vi "Mexa_7170 - 3.vi"(0 "String 1 In":string, 1 "Connect":bool, 2 "IP Array":string[](array[string]), 5 "connection ID 1 In":refnum<k5>, 7 "error out 1 In":errorcluster, 9 "connection ID 2 In":refnum<k16>, 11 "error out 2 In":errorcluster, 12 "Time In":i16) -> (3 "Emissions":dbl[](array[numeric]), 4 "String 1 Out":string, 6 "connection ID 1 Out":refnum<k5>, 8 "error 1 out":errorcluster, 10 "connection ID 2 Out":refnum<k16>, 14 "Time Out":i16, 15 "error 2 out":errorcluster)   [LabVIEW 2014]
panel:
  in  "stop":bool
  out "Array out":dbl[](array[numeric])
  in  "stop TCP 2":bool
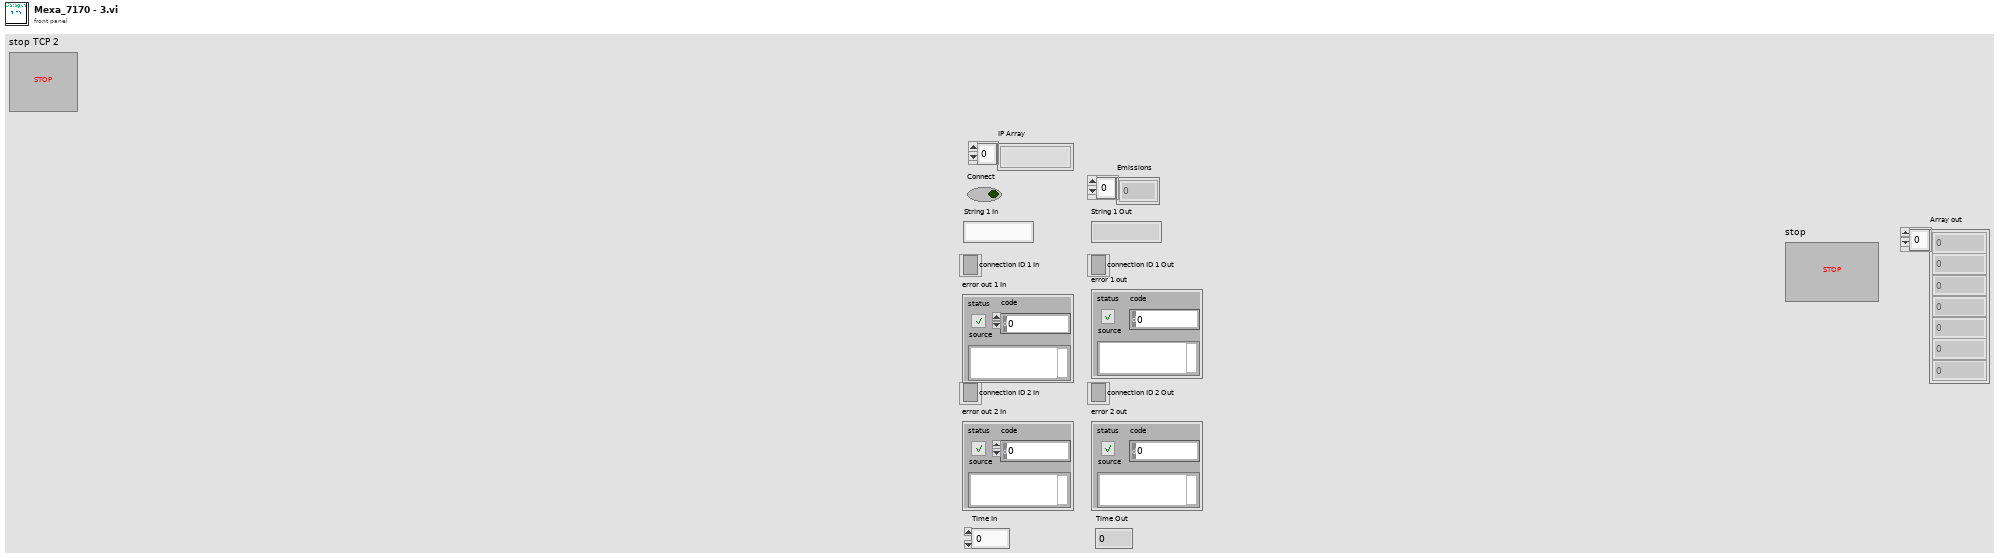
[diagram p1: front panel]
types:
  T1 = cluster{"status":bool, "code":bool, "source":bool}
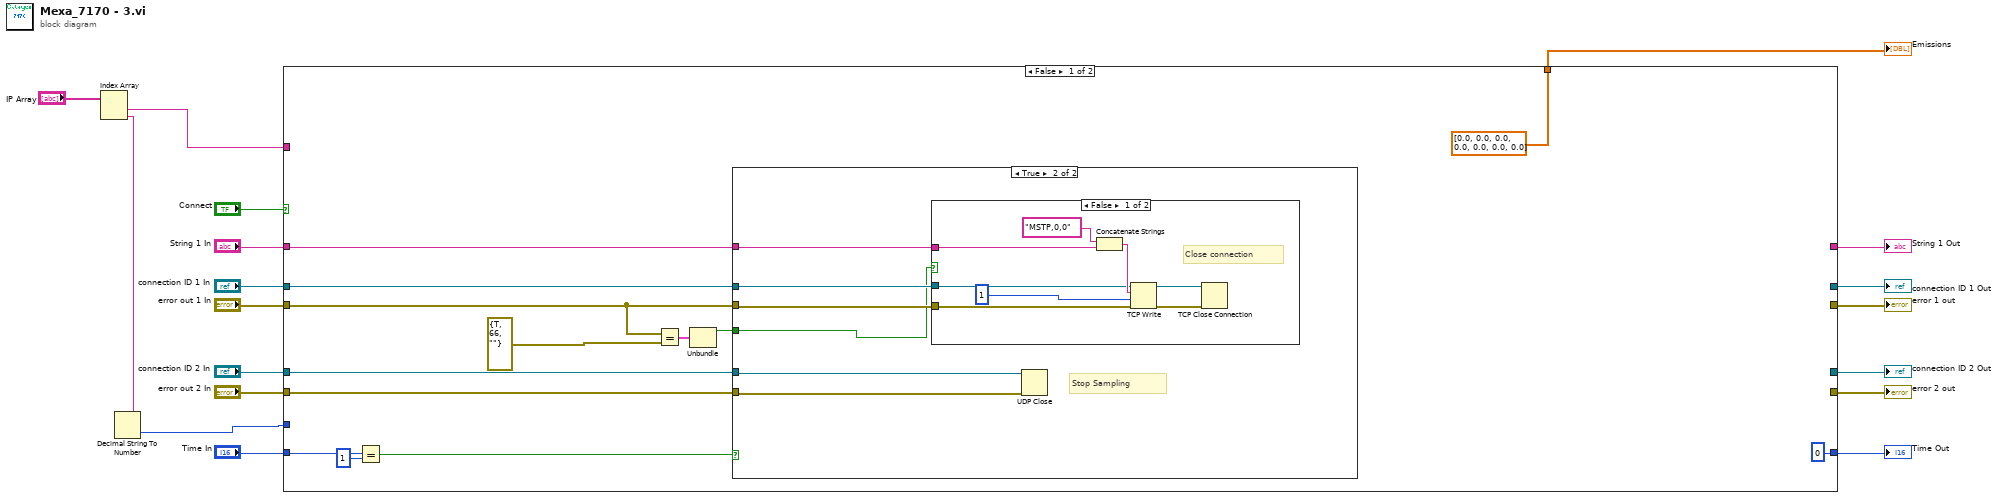
[diagram p0: block diagram]
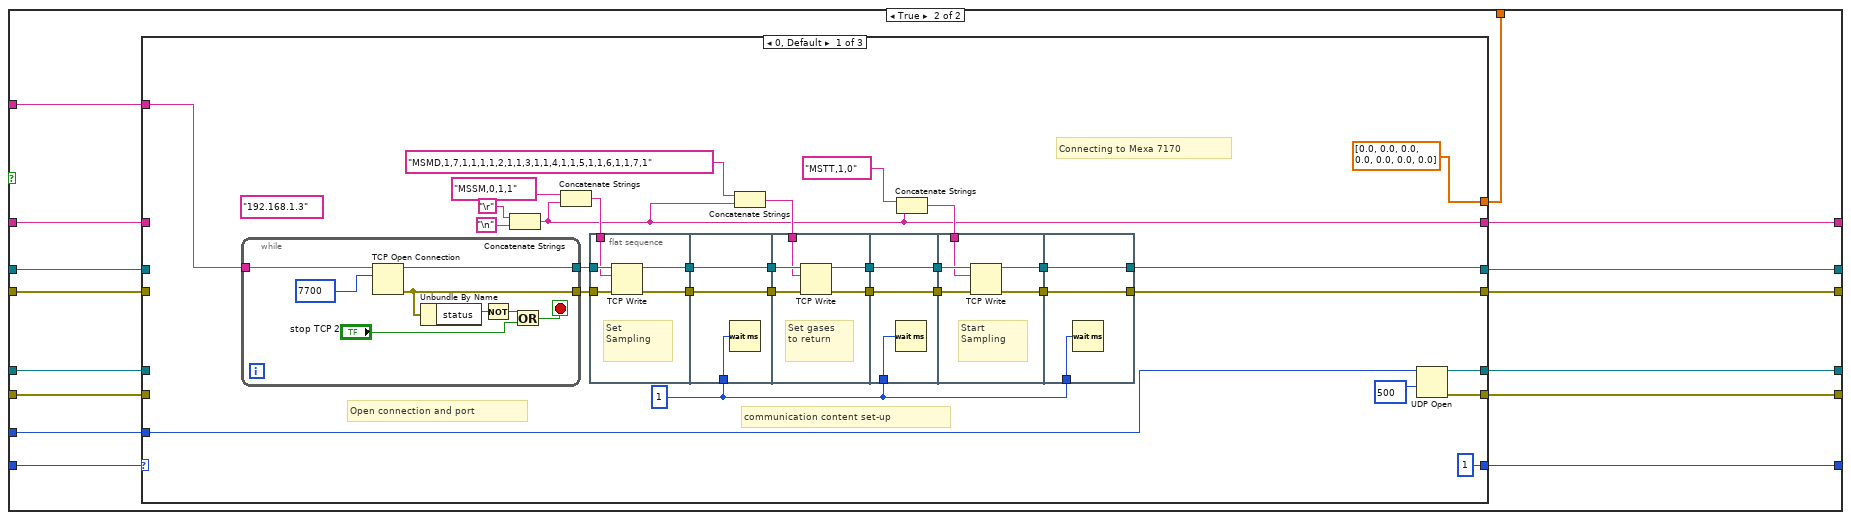
[diagram p4: hidden frame]
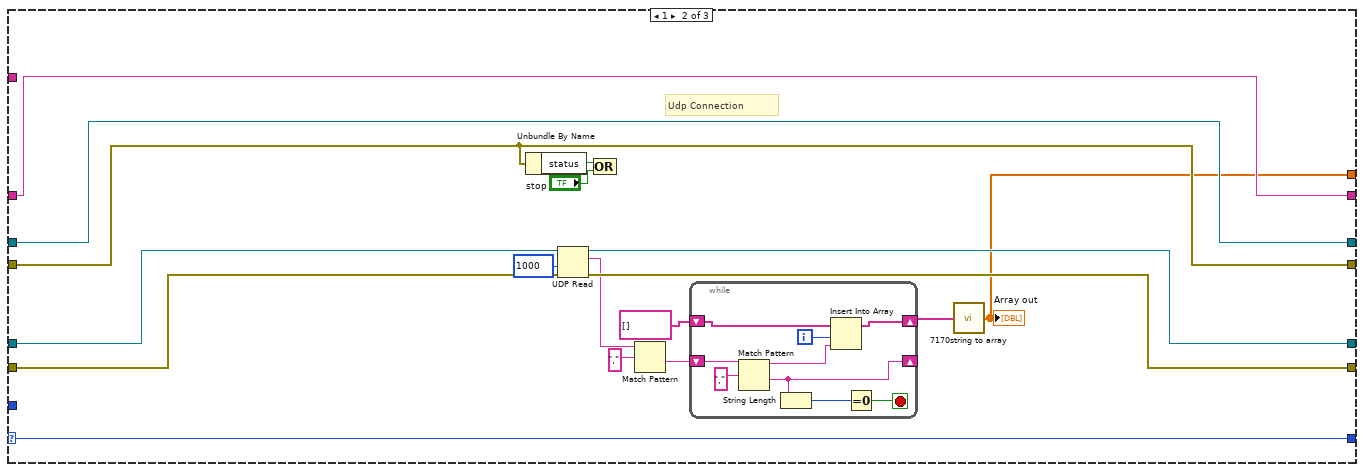
[diagram p5: hidden frame]
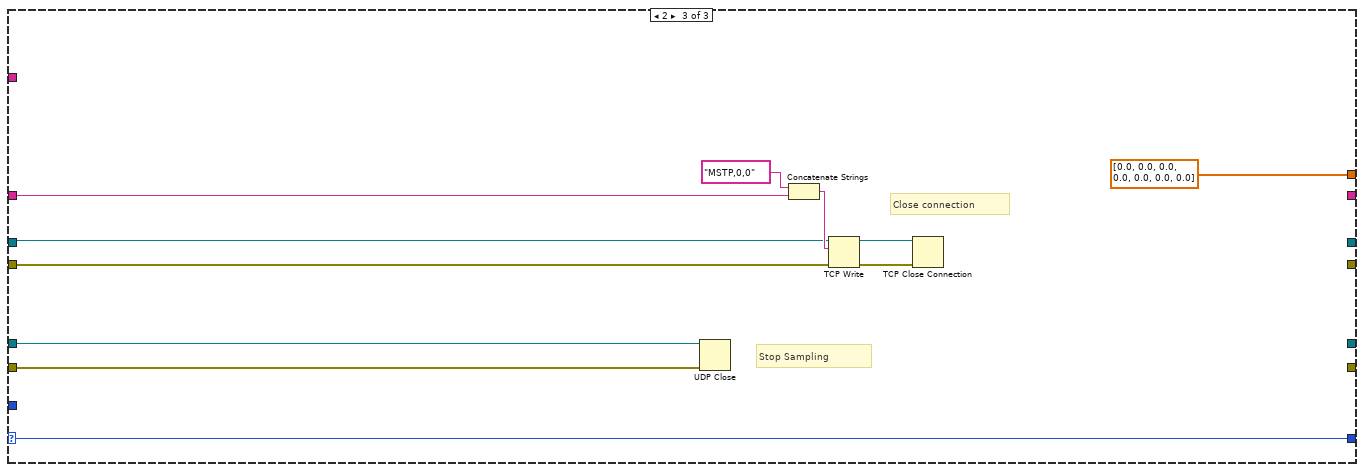
[diagram p6: hidden frame]
diagram:
  n1 = Index Array(array="IP Array") -> (element #1=w3:string, element #2=w1:string)  [unwired: 2 in]
  n2 = Decimal String To Number(string=w1) -> (number=w2:i32)  [unwired: 2 in, 1 out]
  n3 = case shown="False" "Connect" {
    tunnel: [dbl[] [0.0, 0.0, 0.0, 0.0, 0.0, 0.0, 0.0] w60] -> w5
    tunnel: [_ w59] -> w7
    tunnel: [_ w58] -> w8
    tunnel: "connection ID 1 In" -> [w25 w57]
    tunnel: "error out 1 In" -> [w22 w56]
    tunnel: [_ w55] -> w6
    tunnel: "String 1 In" -> [w26 w54]
    tunnel: [_ w53] -> w9
    tunnel: [_ w52] -> w10
    tunnel: "connection ID 2 In" -> [w24 w51]
    tunnel: "error out 2 In" -> [w23 w50]
    tunnel: "Time In" -> [w29 w49]
    tunnel: [i16 0 ("MKS 2") w48] -> w11
    tunnel: w3 -> [_ w47]
    tunnel: w2 -> [_ w46]
    frame False {
      n4 = Equal?(x=w29, y=i16 1) -> (x = y?=w27:bool)
      n5 = Equal?(x=w22, y=errorcluster {"status"=TRUE, "code"=66, "source"=""}) -> (x = y?=w20:T1)
      n6 = Unbundle(w20) -> ("status"=w19:bool)  [unwired: 2 out]
      n7 = case shown="True" w27 {
        tunnel: w26 -> [_ w37]
        tunnel: w25 -> [_ w33]
        tunnel: w22 -> [_ w34]
        tunnel: w24 -> [_ w36]
        tunnel: w23 -> [_ w35]
        tunnel: w19 -> [_ w32]
        frame False {
        }
        frame True {
          # "Stop Sampling"
          n8 = case shown="False" w32 {
            tunnel: w37 -> [w41 _]
            tunnel: w34 -> [w40 _]
            tunnel: w33 -> [w39 _]
            frame False {
              # "Close connection"
              n9 = Concatenate Strings("MSTP,0,0" ("string"), w41) -> (w42:string)
              n10 = TCP Write(connection ID=w39, data in=w42, error in (no error)=w40, 9:1 ("timeout ms (25000)")) -> (connection ID out=w44:refnum<k5>, error out=w45:errorcluster)  [unwired: 1 out]
              n11 = TCP Close Connection(connection ID=w44, error in (no error)=w45) -> ()  [unwired: 1 in, 2 out]
            }
            frame True {
            }
          }
          n12 = UDP Close(connection ID=w36, 8:w35) -> ()  [unwired: 2 out]
        }
      }
    }
    frame True {
      n13 = case shown="0, Default" w49 {
        selector: w49 -> [_ w124 w151]
        tunnel: [dbl[] [0.0, 0.0, 0.0, 0.0, 0.0, 0.0, 0.0] w125 dbl[] [0.0, 0.0, 0.0, 0.0, 0.0, 0.0, 0.0]] -> w60
        tunnel: [w69 w139 _] -> w59
        tunnel: [w68 w138 _] -> w58
        tunnel: w57 -> [_ w139 w156]
        tunnel: w56 -> [_ w138 w155]
        tunnel: [w67 w140 _] -> w55
        tunnel: w54 -> [_ w140 w150]
        tunnel: [w65 w135 _] -> w53
        tunnel: [w64 w134 _] -> w52
        tunnel: w51 -> [_ w137 w154]
        tunnel: w50 -> [_ w136 w153]
        tunnel: [i16 1 ("MKS 2") w124 w151] -> w48
        tunnel: w47 -> [w62 _ _]
        tunnel: w46 -> [w61 _ _]
        frame 0, Default {
          (unwired) "192.168.1.3" ("address")
          w70 = 1
          # "Open connection and port"
          # "communication content set-up"
          # "Connecting to Mexa 7170"
          n14 = while {
            tunnel: [w121] -> w80
            tunnel: [w120] -> w79
            tunnel: w62 -> [w116]
            stop <- w117 stop-if-true
            n15 = TCP Open Connection(address=w116, remote port or service name=u16 7700) -> (connection ID=w121:refnum<k5>, error out=w120:errorcluster)  [unwired: 3 in]
            n16 = Unbundle By Name(w120) -> ("status"=w122:bool)
            n17 = Not(x=w122) -> (.not. x?=w118:bool)
            n18 = Or(x=w118, y="stop TCP 2") -> (x .or. y?=w117:bool)
          }
          n19 = Concatenate Strings("\r", "\n") -> (w67:string)
          n20 = Concatenate Strings("MSSM,0,1,1" ("data in"), w67) -> (w75:string)
          n21 = flat-sequence {
            tunnel: w80 -> [w96]
            tunnel: w79 -> [w95]
            tunnel: w75 -> [w94]
            tunnel: [w93] -> w90
            tunnel: [w92] -> w89
            tunnel: w90 -> [w99]
            tunnel: w89 -> [w98]
            tunnel: w70 -> [w97]
            tunnel: [w99] -> w88
            tunnel: [w98] -> w87
            tunnel: w88 -> [w103]
            tunnel: w87 -> [w104]
            tunnel: w72 -> [w102]
            tunnel: [w100] -> w86
            tunnel: [w101] -> w85
            tunnel: w86 -> [w107]
            tunnel: w85 -> [w106]
            tunnel: w70 -> [w105]
            tunnel: [w107] -> w84
            tunnel: [w106] -> w83
            tunnel: w84 -> [w111]
            tunnel: w83 -> [w112]
            tunnel: w71 -> [w108]
            tunnel: [w110] -> w82
            tunnel: [w109] -> w81
            tunnel: [w114] -> w69
            tunnel: [w115] -> w68
            tunnel: w82 -> [w115]
            tunnel: w81 -> [w114]
            tunnel: w70 -> [w113]
            frame #0 {
              # "Set \nSampling"
              n22 = TCP Write(connection ID=w96, data in=w94, error in (no error)=w95) -> (connection ID out=w92:refnum<k5>, error out=w93:errorcluster)  [unwired: 1 in, 1 out]
            }
            frame #1 {
              n23 = Wait (ms)(milliseconds to wait=w97) -> ()  [unwired: 1 out]
            }
            frame #2 {
              # "Set gases\nto return"
              n24 = TCP Write(connection ID=w104, data in=w102, error in (no error)=w103) -> (connection ID out=w101:refnum<k5>, error out=w100:errorcluster)  [unwired: 1 in, 1 out]
            }
            frame #3 {
              n25 = Wait (ms)(milliseconds to wait=w105) -> ()  [unwired: 1 out]
            }
            frame #4 {
              # "Start\nSampling"
              n26 = TCP Write(connection ID=w112, data in=w108, error in (no error)=w111) -> (connection ID out=w109:refnum<k5>, error out=w110:errorcluster)  [unwired: 1 in, 1 out]
            }
            frame #5 {
              n27 = Wait (ms)(milliseconds to wait=w113) -> ()  [unwired: 1 out]
            }
          }
          n28 = Concatenate Strings("MSMD,1,7,1,1,1,1,2,1,1,3,1,1,4,1,1,5,1,1,6,1,1,7,1" ("data in"), w67) -> (w72:string)
          n29 = Concatenate Strings("MSTT,1,0" ("string"), w67) -> (w71:string)
          n30 = UDP Open(9:500 ("timeout ms (25000)"), 11:w61) -> (port=w65:refnum<k16>, 0:w64:errorcluster)  [unwired: 3 in, 1 out]
        }
        frame 1 {
          # "Udp Connection"
          n31 = Unbundle By Name(w138) -> ("status"=w132:bool)
          n32 = UDP Read(connection ID=w137, timeout ms (25000)=1000, 8:w136) -> (data out=w128:string, error out=w134:errorcluster, 3:w135:refnum<k16>)  [unwired: 1 in, 2 out]
          n33 = Compound Arithmetic op=OR(w132, "stop") -> ()  [unwired: 1 out]
          n34 = Match Pattern(string=w128, regular expression="," ("search string/char (-)")) -> (after substring=w129:string)  [unwired: 1 in, 3 out]
          n35 = while {
            shift-right: [w145] -> w126
            shift-left: string[] [] -> [w146]
            shift-right: [w144] -> _
            shift-left: w129 -> [w148]
            i -> [w143]
            stop <- w142 stop-if-true
            n36 = Match Pattern(string=w148, regular expression="," ("search string/char (-)")) -> (before substring=w147:string, after substring=w144:string)  [unwired: 1 in, 2 out]
            n37 = String Length(string=w144) -> (length=w141:i32)
            n38 = Insert Into Array(array=w146, index=w143, new element=w147) -> (w145:string[])
            n39 = Equal To 0?(x=w141) -> (x = 0?=w142:bool)
          }
          n40 = call "7170string to array.vi"("Array in"=w126) -> ("Array out"=w125:dbl[])  [unwired: 4 in]
          "Array out" <- w125
        }
        frame 2 {
          # "Close connection"
          # "Stop Sampling"
          n41 = UDP Close(connection ID=w154, 8:w153) -> ()  [unwired: 2 out]
          n42 = Concatenate Strings("MSTP,0,0" ("string"), w150) -> (w157:string)
          n43 = TCP Write(connection ID=w156, data in=w157, error in (no error)=w155) -> (connection ID out=w159:refnum<k5>, error out=w160:errorcluster)  [unwired: 1 in, 1 out]
          n44 = TCP Close Connection(connection ID=w159, error in (no error)=w160) -> ()  [unwired: 1 in, 2 out]
        }
      }
    }
  }
  "Time Out" <- w11
  "error 2 out" <- w10
  "connection ID 2 Out" <- w9
  "error 1 out" <- w8
  "connection ID 1 Out" <- w7
  "String 1 Out" <- w6
  "Emissions" <- w5
